vi "Control Multiple Analog Outputs - Static.vi"(0 "Line":tag="Dev1/port0/line0:7", 5 "Voltage":dbl[](array[numeric]), 11 "Error In":errorcluster) -> (15 "Error Out":errorcluster)   [LabVIEW 2016]
doc: "This VI generates a static analog voltage output on the line you specify."
uses:
  <vilib>/DAQmx/write.llb/DAQmx Write (Analog 1D DBL NChan 1Samp).vi
  <vilib>/DAQmx/create/channels.llb/DAQmx Create Channel (AO-Voltage-Basic).vi
  <vilib>/DAQmx/miscellaneous.llb/DAQmx Fill In Error Info.vi
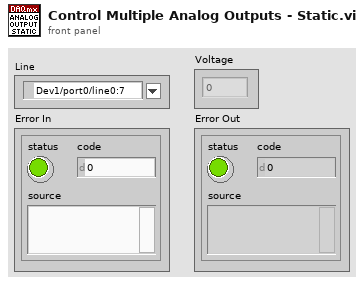
[diagram p1: front panel]
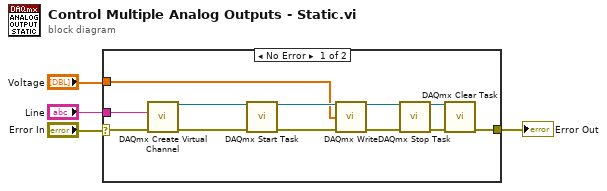
[diagram p0: block diagram]
diagram:
  n1 = case shown="No Error" "Error In" {
    selector: "Error In" -> [w8 w17]
    tunnel: "Line" -> [w7 _]
    tunnel: "Voltage" -> [w6 _]
    tunnel: [w5 w17] -> w2
    frame No Error {
      n2 = call-poly <vilib>:"DAQmx Create Virtual Channel.vi"("physical channels"=w7, "error in"=w8) -> ("task out"=w13:refnum<k21>, "error out"=w14:errorcluster)  [unwired: 12 in]
      n3 = call <vilib>:"DAQmx Start Task.vi"("task/channels in"=w13, "error in"=w14) -> ("task out"=w16:refnum<k21>, "error out"=w15:errorcluster)  [unwired: 12 in]
      n4 = call-poly <vilib>:"DAQmx Write.vi"("task/channels in"=w16, "data"=w6, "error in"=w15) -> ("task out"=w10:refnum<k21>, "error out"=w9:errorcluster)  [unwired: 10 in, 1 out]
      n5 = call <vilib>:"DAQmx Stop Task.vi"("task/channels in"=w10, "error in"=w9) -> ("task out"=w12:refnum<k21>, "error out"=w11:errorcluster)  [unwired: 12 in]
      n6 = call <vilib>:"DAQmx Clear Task.vi"("task in"=w12, "error in"=w11) -> ("error out"=w5:errorcluster)  [unwired: 13 in]
    }
    frame Error {
    }
  }
  "Error Out" <- w2
